vi "Adjust dB to Vbias Gain Words.vi"(11 "Adjust dB":dbl) -> (2 "Vbias Word":u8 format="%.0b", 3 "Gain Word":u8 format="%.0b")   [LabVIEW 2020]
panel:
  out "Gain Word Axis":u8[](array[numeric])
  out "Vbias Word Axis":u8[](array[numeric])
  out "Gain dB Axis":dbl[](array[numeric])
  out "Vbias dB Axis":dbl[](array[numeric])
  out "Error (dB)":dbl[][](array[numeric])
  out "Vbias Gain dB":dbl
  out "Gain dB":dbl
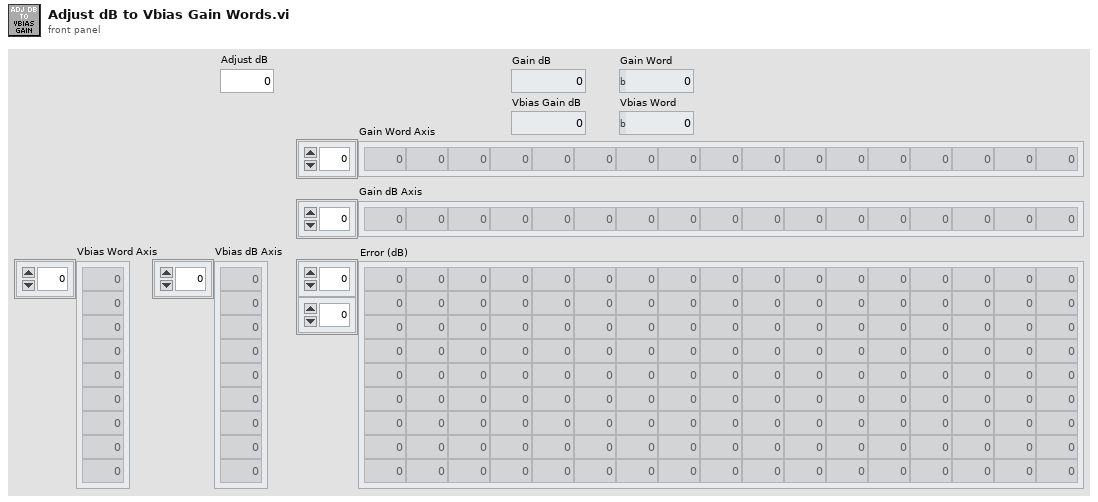
[diagram p1: front panel]
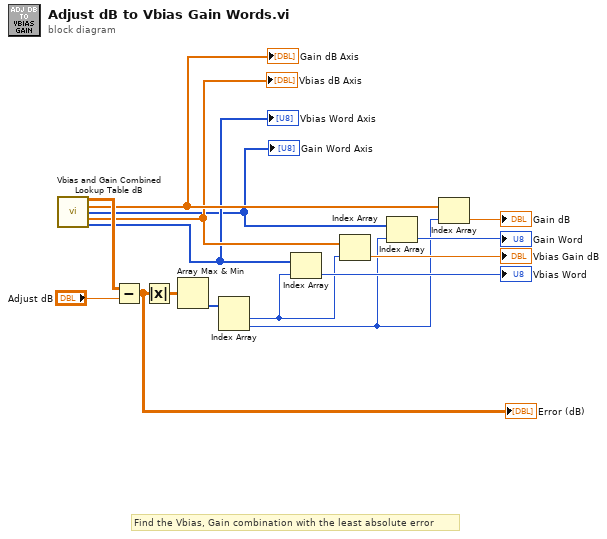
[diagram p0: block diagram]
diagram:
  # "Find the Vbias, Gain combination with the least absolute error"
  n1 = call "Vbias and Gain Combined Lookup Table dB.vi"() -> ("Vbias vs Gain combined dB"=w15:dbl[][], "Gain dB"=w4:dbl[], "Gain Word"=w1:u8[], "Vbias dB"=w3:dbl[], "Vbias Word"=w2:u8[])  [unwired: 11 in]
  "Vbias dB Axis" <- w3
  "Gain dB Axis" <- w4
  "Vbias Word Axis" <- w2
  "Gain Word Axis" <- w1
  n2 = Subtract(x=w15, y="Adjust dB") -> (x-y=w13:dbl[][])
  "Error (dB)" <- w13
  n3 = Absolute Value(x=w13) -> (abs(x)=w12:dbl[][])
  n4 = Array Max & Min(array=w12) -> (min index (indices)=w11:i32[])  [unwired: 3 out]
  n5 = Index Array(array=w11) -> (element #1=w6:i32, element #2=w5:i32)  [unwired: 2 in]
  n6 = Index Array(array=w2, index=w6) -> (element=→"Vbias Word":u8)
  n7 = Index Array(array=w3, index=w6) -> (element=→"Vbias Gain dB":dbl)
  n8 = Index Array(array=w1, index=w5) -> (element=→"Gain Word":u8)
  n9 = Index Array(array=w4, index=w5) -> (element=→"Gain dB":dbl)
